vi "进度条演示.vi"() -> ()   [LabVIEW 2020]
panel:
  out "滑动杆进度条":dbl(slide) scale=0.0..1.0
  out "文件名":string
  in  "路径":path
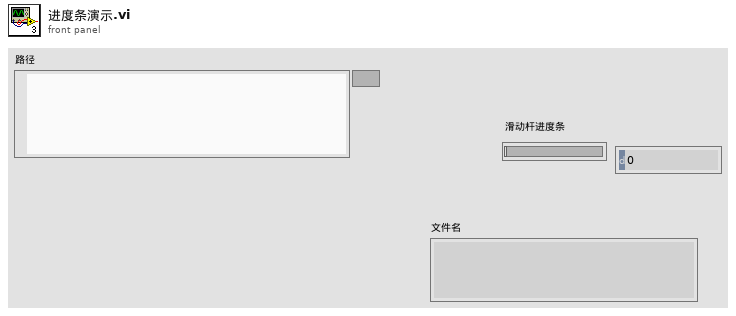
[diagram p1: front panel]
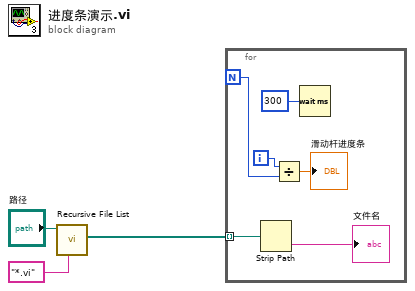
[diagram p0: block diagram]
diagram:
  n1 = call <vilib>:"Recursive File List.vi"("pattern"="*.vi", "Folder Path"="路径") -> ("All Files in Dir"=w1:path[])  [unwired: 5 in, 4 out]
  n2 = for {
    N -> [w8]
    tunnel: w1 -> [w7] mode=indexing
    i -> [w9]
    n3 = Strip Path(path=w7) -> (name=→"文件名":string)  [unwired: 1 out]
    n4 = Divide(x=w9, y=w8) -> (x/y=→"滑动杆进度条":dbl)
    n5 = Wait (ms)(milliseconds to wait=300) -> ()  [unwired: 1 out]
  }
